vi "lectura_motion.vi"(10 "Address Type":T1=1 items=["Public", "Random"], 11 "COM Bluegiga in":refnum<visa-resource-name>="COM13") -> (3 "Connected":bool)   [LabVIEW 2020]
uses:
  <vilib>/BLE/type_def/connection_status_bundle.ctl
  <vilib>/BLE/type_def/address_type.ctl
panel:
  out "Count":u8
  out "Z DOWN":bool
  out "Z UP":bool
  out "Y DOWN":bool
  out "Y UP":bool
  out "X DOWN":bool
  out "X UP":bool
  out "Numeric":dbl
  out "Text":string caption="Result"
  out "z 4":dbl
  out "y 4":dbl
  out "x 4":dbl
  out "w 4":dbl
  in  "stop":bool
  in  "Array":string[][](array[string])
  out "MAC Address":string
  out "Handle table":string[][](array[string])
  out "Connection Status":T2={"MAC Address"="", "cnx handle"=0, "cnx flags"=0, "Address Type"=125, "Connection Interval (ms)"=125, "Timeout(ms)"=125, "Latency"=0, "bonding handle"=0} {"Address Type" items=["Public", "Random"]}
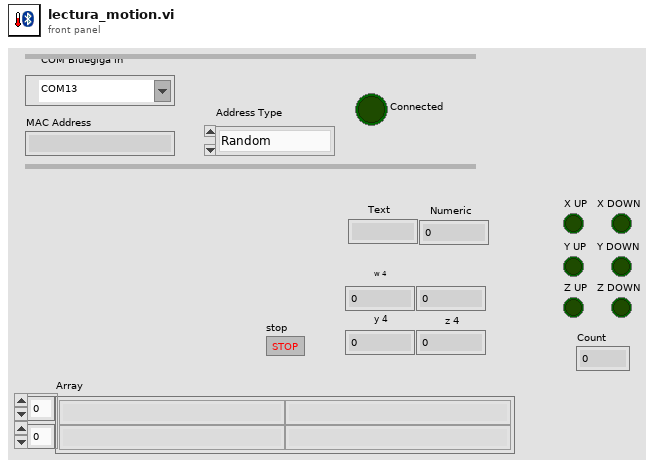
[diagram p1: front panel]
types:
  T1 = typedef "address_type.ctl" = u8
  T2 = typedef "connection_status_bundle.ctl" = cluster{"MAC Address":string, "cnx handle":u8, "cnx flags":u8, "Address Type":T1, "Connection Interval (ms)":u16, "Timeout(ms)":u16, "Latency":u16, "bonding handle":u8}
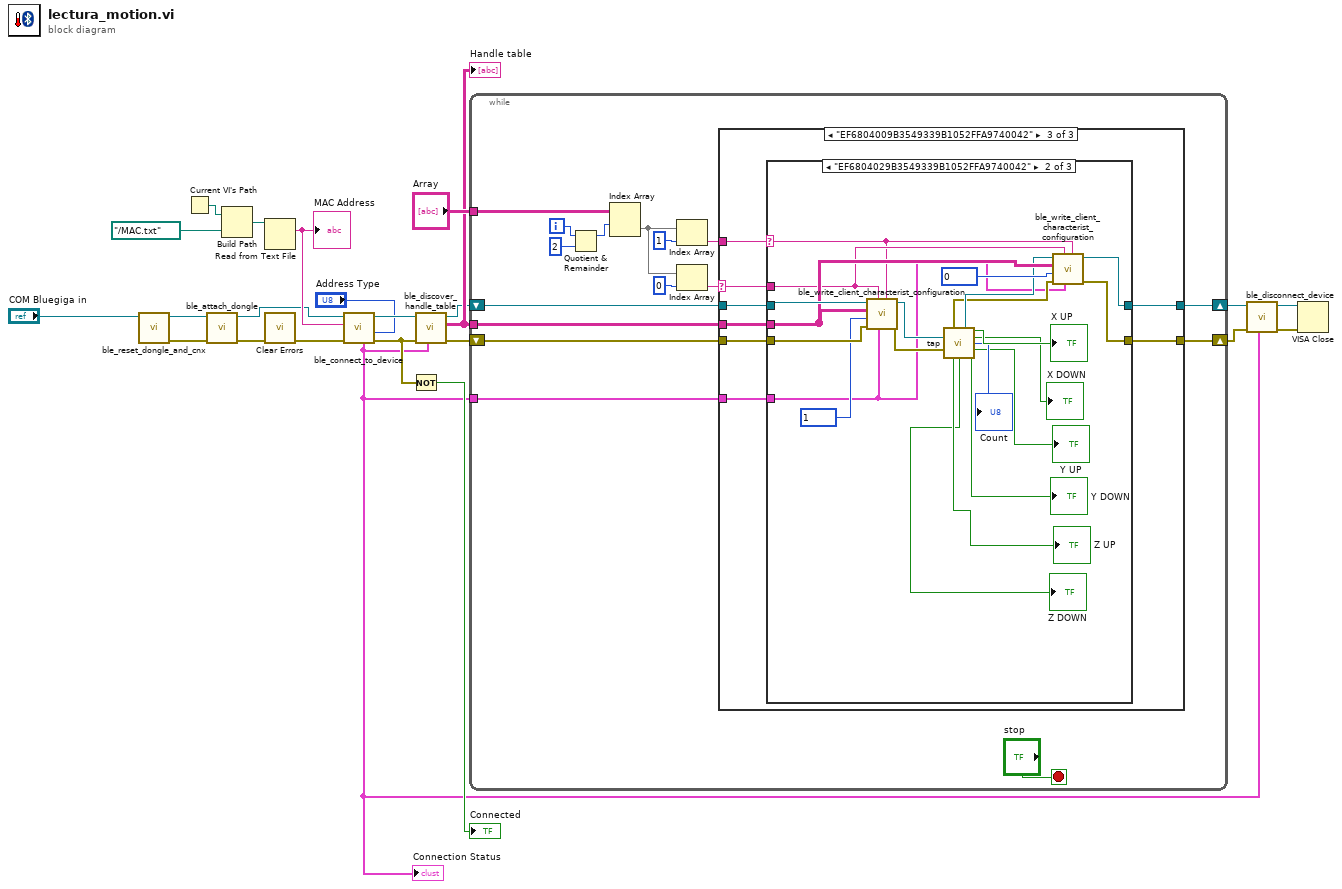
[diagram p0: block diagram]
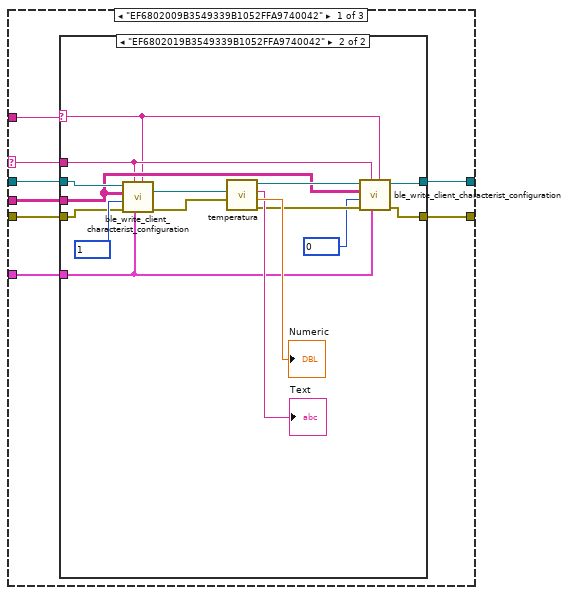
[diagram p2: hidden frame]
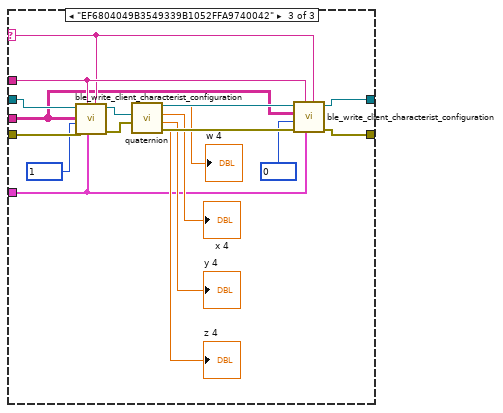
[diagram p6: hidden frame]
diagram:
  n1 = call <vilib>:"ble_reset_dongle_and_cnx.vi"("COM Bluegiga in"="COM Bluegiga in") -> ("error out"=w21:errorcluster, "COM Bluegiga out"=w19:refnum<visa-resource-name>)  [unwired: 9 in]
  n2 = Current VI's Path() -> (path=w11:path)
  n3 = call <vilib>:"ble_attach_dongle.vi"("error in (no error)"=w21, "COM Bluegiga in"=w19) -> ("error out"=w9:errorcluster, "COM Bluegiga out"=w10:refnum<visa-resource-name>)  [unwired: 8 in]
  n4 = Build Path(base path=w11, name or relative path=path "../MAC.txt") -> (appended path=w12:path)
  n5 = Read from Text File(file (use dialog)=w12) -> (text=w14:string)  [unwired: 3 in, 3 out]
  "MAC Address" <- w14
  n6 = call <vilib>:"Clear Errors.vi"("error in (no error)"=w9) -> ("error out"=w16:errorcluster)  [unwired: 5 in, 1 out]
  n7 = call <vilib>:"ble_connect_to_device.vi"("Address Type"="Address Type", "error in (no error)"=w16, "MAC Address"=w14, "COM Bluegiga in"=w10) -> ("error out"=w17:errorcluster, "COM Bluegiga out"=w18:refnum<visa-resource-name>, "Connection Status"=w4:T2)  [unwired: 5 in]
  "Connection Status" <- w4
  n8 = Not(x=w17) -> (.not. x?=→"Connected":bool)
  n9 = call <vilib>:"ble_discover_handle_table.vi"("Connection Status"=w4, "error in (no error)"=w17, "COM Bluegiga in"=w18) -> ("error out"=w2:errorcluster, "Handle table"=w3:string[][], "COM Bluegiga out"=w1:refnum<visa-resource-name>)  [unwired: 6 in]
  "Handle table" <- w3
  n10 = while {
    tunnel: "Array" -> [w30]
    shift-right: [w36] -> w5
    shift-left: w2 -> [w39]
    shift-right: [w37] -> w6
    shift-left: w1 -> [w38]
    tunnel: w4 -> [w35]
    tunnel: w3 -> [w34]
    i -> [w33]
    stop <- "stop" stop-if-true
    n11 = Quotient & Remainder(x=w33, y=2) -> (x-y*floor(x/y)=w29:i32)  [unwired: 1 out]
    n12 = Index Array(array=w30, index (row)=w29) -> (element=w28:string[])  [unwired: 1 in]
    n13 = Index Array(array=w28, index=1) -> (element=w24:string)
    n14 = Index Array(array=w28, index=0) -> (element=w25:string)
    n15 = case shown="\"EF6804009B3549339B1052FFA9740042\"" w25 {
      selector: w25 -> [w46 _ w68]
      tunnel: w39 -> [w43 w66 w73]
      tunnel: w38 -> [w45 w67 w74]
      tunnel: [w41 w67 w71] -> w37
      tunnel: [w40 w66 w70] -> w36
      tunnel: w35 -> [w42 _ w72]
      tunnel: w34 -> [w44 _ w69]
      tunnel: w24 -> [w47 _ w75]
      frame "EF6802009B3549339B1052FFA9740042" {
        n16 = case shown="\"EF6802019B3549339B1052FFA9740042\"" w47 {
          selector: w47 -> [_ w50]
          tunnel: w46 -> [_ w51]
          tunnel: w45 -> [w49 w57]
          tunnel: w44 -> [_ w55]
          tunnel: w43 -> [w48 w56]
          tunnel: w42 -> [_ w54]
          tunnel: [w49 w52] -> w41
          tunnel: [w48 w53] -> w40
          frame Default {
          }
          frame "EF6802019B3549339B1052FFA9740042" {
            n17 = call <vilib>:"ble_write_client_characterist_configuration.vi"("Characteristic UUID"=w50, "Connection Status"=w54, "Service UUID"=w51, "error in (no error)"=w56, "Value(16bit)"=u16 1, "Handle table"=w55, "COM Bluegiga in"=w57) -> ("error out"=w63:errorcluster, "COM Bluegiga out"=w62:refnum<visa-resource-name>)  [unwired: 3 in]
            n18 = call "temperatura.vi"("error in (no error)"=w63, "COM Bluegiga in"=w62) -> ("error out"=w61:errorcluster, "Numeric"=→"Numeric":dbl, "Text"=→"Text":string, "COM Bluegiga out"=w60:refnum<visa-resource-name>)  [unwired: 6 in]
            n19 = call <vilib>:"ble_write_client_characterist_configuration.vi"("Characteristic UUID"=w50, "Connection Status"=w54, "Service UUID"=w51, "error in (no error)"=w61, "Value(16bit)"=u16 0, "Handle table"=w55, "COM Bluegiga in"=w60) -> ("error out"=w53:errorcluster, "COM Bluegiga out"=w52:refnum<visa-resource-name>)  [unwired: 3 in]
          }
        }
      }
      frame Default {
      }
      frame "EF6804009B3549339B1052FFA9740042" {
        n20 = case shown="\"EF6804029B3549339B1052FFA9740042\"" w75 {
          selector: w75 -> [_ w79 w103]
          tunnel: w74 -> [w77 w87 w106]
          tunnel: w73 -> [w76 w91 w107]
          tunnel: w72 -> [_ w78 w101]
          tunnel: [w77 w81 w100] -> w71
          tunnel: [w76 w82 w99] -> w70
          tunnel: w69 -> [_ w85 w102]
          tunnel: w68 -> [_ w80 w104]
          frame Default {
          }
          frame "EF6804029B3549339B1052FFA9740042" {
            n21 = call <vilib>:"ble_write_client_characterist_configuration.vi"("Characteristic UUID"=w79, "Connection Status"=w78, "Service UUID"=w80, "error in (no error)"=w91, "Value(16bit)"=u16 1, "Handle table"=w85, "COM Bluegiga in"=w87) -> ("error out"=w88:errorcluster, "COM Bluegiga out"=w89:refnum<visa-resource-name>)  [unwired: 3 in]
            n22 = call "tap.vi"("COM Bluegiga in"=w89, "error in (no error)"=w88) -> ("error out"=w83:errorcluster, "COM Bluegiga out"=w84:refnum<visa-resource-name>, "X UP"=→"X UP":bool, "X DOWN"=→"X DOWN":bool, "Count"=→"Count":u8, "Y UP"=→"Y UP":bool, "Z UP"=→"Z UP":bool, "Z DOWN"=→"Z DOWN":bool, "Y DOWN"=→"Y DOWN":bool)  [unwired: 5 in]
            n23 = call <vilib>:"ble_write_client_characterist_configuration.vi"("Characteristic UUID"=w79, "Connection Status"=w78, "Service UUID"=w80, "error in (no error)"=w83, "Value(16bit)"=u16 0, "Handle table"=w85, "COM Bluegiga in"=w84) -> ("error out"=w82:errorcluster, "COM Bluegiga out"=w81:refnum<visa-resource-name>)  [unwired: 3 in]
          }
          frame "EF6804049B3549339B1052FFA9740042" {
            n24 = call <vilib>:"ble_write_client_characterist_configuration.vi"("Characteristic UUID"=w103, "Connection Status"=w101, "Service UUID"=w104, "error in (no error)"=w107, "Value(16bit)"=u16 1, "Handle table"=w102, "COM Bluegiga in"=w106) -> ("error out"=w114:errorcluster, "COM Bluegiga out"=w113:refnum<visa-resource-name>)  [unwired: 3 in]
            n25 = call "quaternion.vi"("error in (no error)"=w114, "COM Bluegiga in"=w113) -> ("z"=→"z 4":dbl, "y"=→"y 4":dbl, "x"=→"x 4":dbl, "w"=→"w 4":dbl, "COM Bluegiga out"=w115:refnum<visa-resource-name>, "error out"=w116:errorcluster)  [unwired: 4 in]
            n26 = call <vilib>:"ble_write_client_characterist_configuration.vi"("Characteristic UUID"=w103, "Connection Status"=w101, "Service UUID"=w104, "error in (no error)"=w116, "Value(16bit)"=u16 0, "Handle table"=w102, "COM Bluegiga in"=w115) -> ("error out"=w99:errorcluster, "COM Bluegiga out"=w100:refnum<visa-resource-name>)  [unwired: 3 in]
          }
        }
      }
    }
  }
  n27 = call <vilib>:"ble_disconnect_device.vi"("Connection Status"=w4, "error in (no error)"=w5, "COM Bluegiga in"=w6) -> ("error out"=w22:errorcluster, "COM Bluegiga out"=w23:refnum<visa-resource-name>)  [unwired: 7 in]
  n28 = VISA Close(VISA resource name=w23, error in (no error)=w22) -> ()  [unwired: 1 out]
